vi "getActionPanelPath.vi"(8 "error in (no error)":errorcluster, 11 "ChangeValueAction in":refnum<class "ChangeValueAction.lvclass">) -> (0 "error out":errorcluster, 2 "frontPanelPath":path, 3 "ChangeValueAction out":refnum<class "ChangeValueAction.lvclass">)   [LabVIEW 2011, in "Views.lvlib" / "ScriptEditor.lvlib" / "ChangeValueAction.lvclass"]
uses:
  ChangeValueAction.lvclass
  Tools/Filing/FileSystem/FileSystem.lvclass
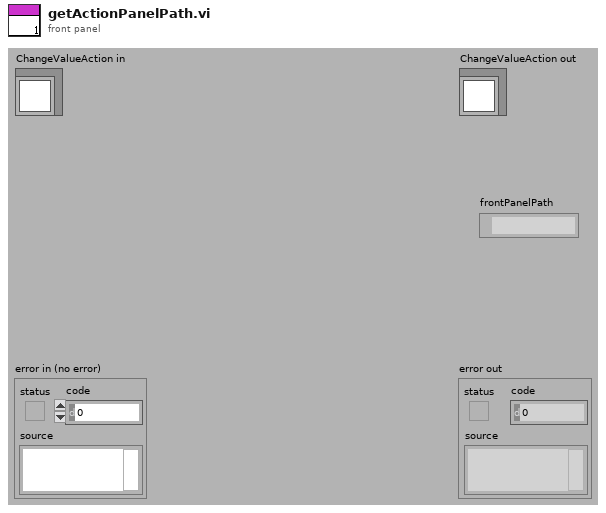
[diagram p1: front panel]
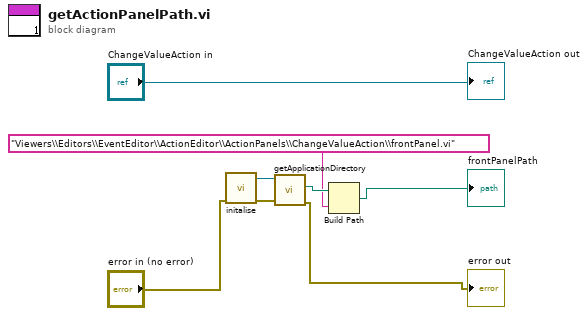
[diagram p0: block diagram]
diagram:
  n1 = call "initalise.vi"("error in (no error)"="error in (no error)") -> ("error out"=w8:errorcluster, "FileSystem out"=w7:refnum<class "FileSystem.lvclass">)  [unwired: 9 in]
  n2 = call-dynamic "getApplicationDirectory.vi"("error in (no error)"=w8, "FileSystem.lvclass in"=w7) -> ("error out"=→"error out":errorcluster, "ApplicationDirectory"=w5:path)  [unwired: 7 in, 1 out]
  n3 = Build Path(base path=w5, name or relative path="Viewers\\Editors\\EventEditor\\ActionEditor\\ActionPanels\\ChangeValueAction\\frontPanel.vi") -> (appended path=→"frontPanelPath":path)
  "ChangeValueAction out" <- "ChangeValueAction in"
